vi "calculate_detection_gates.vi"(9 "gates_calculation":enum16{"Software", "Hardware"}(ring), 10 "triggers":u32[][](array[numeric]), 11 "T1_parameters":T1) -> (2 "start_read":u32[][](array[numeric]), 3 "stop_read":u32[][](array[numeric]))   [LabVIEW 2018]
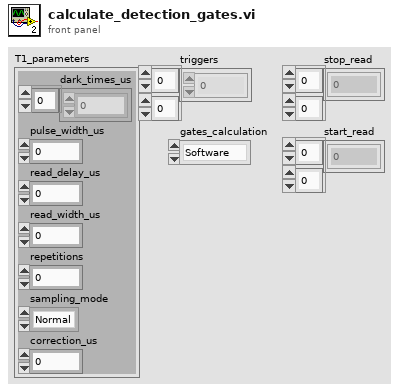
[diagram p1: front panel]
types:
  T1 = cluster{"dark_times_us":dbl[], "pulse_width_us":dbl, "read_delay_us":dbl, "read_width_us":dbl, "repetitions":i32, "sampling_mode":enum16{"Normal", "Sweep"}, "correction_us":dbl}
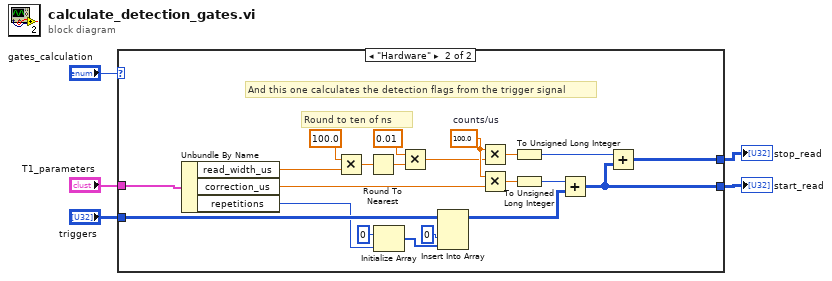
[diagram p0: block diagram]
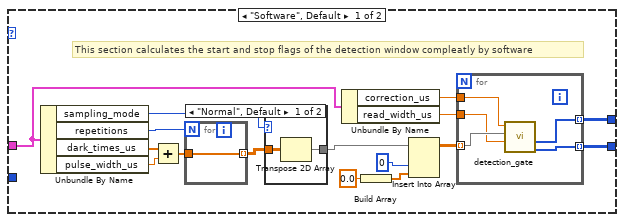
[diagram p2: hidden frame]
diagram:
  n1 = case shown="\"Hardware\"" "gates_calculation" {
    tunnel: "T1_parameters" -> [w8 w45]
    tunnel: "triggers" -> [_ w40]
    tunnel: [w7 w31] -> w2
    tunnel: [w6 w32] -> w1
    frame "Software", Default {
      # "This section calculates the start and stop flags of the detection window compleatly by software"
      n2 = Unbundle By Name(w8) -> ("sampling_mode"=w16:enum16{"Normal", "Sweep"}, "repetitions"=w19:i32, "dark_times_us"=w20:dbl[], "pulse_width_us"=w21:dbl)
      n3 = Add(x=w20, y=w21) -> (x+y=w18:dbl[])
      n4 = for {
        N: w19 -> [_]
        tunnel: [w30] -> w17 mode=indexing
        tunnel: w18 -> [w30]
      }
      n5 = case shown="\"Normal\", Default" w16 {
        tunnel: w17 -> [w27 w29]
        tunnel: [w28 w29] -> w15
        frame "Normal", Default {
          n6 = Transpose 2D Array(2D array=w27) -> (transposed array=w28:dbl[][])
        }
        frame "Sweep" {
        }
      }
      n7 = Unbundle By Name(w8) -> ("correction_us"=w11:dbl, "read_width_us"=w10:dbl)
      n8 = Build Array(0.0 ("element")) -> (w12:dbl[])
      n9 = Insert Into Array(array=w15, index (col)=0 ("disabled index (col)"), new element=w12) -> (w9:dbl[][])  [unwired: 1 in]
      n10 = for {
        tunnel: w9 -> [w26] mode=indexing
        tunnel: w11 -> [w24]
        tunnel: w10 -> [w25]
        tunnel: [w23] -> w7 mode=indexing
        tunnel: [w22] -> w6 mode=indexing
        n11 = call "detection_gate.vi"("read_width_us"=w25, "pulse_period_us"=w26, "correction_us"=w24) -> ("start_read"=w22:u32[], "stop_read"=w23:u32[])  [unwired: 7 in]
      }
    }
    frame "Hardware" {
      w51 = 100.0  # counts/us
      # "Round to ten of ns"
      # "And this one calculates the detection flags from the trigger signal"
      n12 = Unbundle By Name(w45) -> ("read_width_us"=w50:dbl, "correction_us"=w44:dbl, "repetitions"=w36:i32)
      n13 = Multiply(x=100.0, y=w50) -> (x*y=w46:dbl)
      n14 = Round To Nearest(number=w46) -> (nearest integer value=w47:dbl)
      n15 = Initialize Array(0 ("index (row)"), w36) -> (w39:i32[])
      n16 = Multiply(x=0.01, y=w47) -> (x*y=w43:dbl)
      n17 = Insert Into Array(array=w40, index (col)=0 ("index (row)"), new element=w39) -> (w35:u32[][])  [unwired: 1 in]
      n18 = Multiply(x=w51, y=w43) -> (x*y=w42:dbl)
      n19 = Multiply(x=w51, y=w44) -> (x*y=w41:dbl)
      n20 = To Unsigned Long Integer(number=w42) -> (unsigned 32bit integer=w33:u32)
      n21 = To Unsigned Long Integer(number=w41) -> (unsigned 32bit integer=w34:u32)
      n22 = Add(x=w34, y=w35) -> (x+y=w32:u32[][])
      n23 = Add(x=w33, y=w32) -> (x+y=w31:u32[][])
    }
  }
  "stop_read" <- w2
  "start_read" <- w1
